vi "Write Permissions.vi"(8 "Error In":errorcluster) -> (0 "Error Out":errorcluster)   [LabVIEW 2018, in "Tests.lvlib" / "SFTP Attributes.lvlib"]
uses:
  SFTP Attributes.lvlib
  src/Toolkit/API/Typedefs/Permissions.ctl
  src/Toolkit/API/Typedefs/Modes.ctl
  src/Toolkit/API/SFTP Attributes/SFTP Attributes.lvclass/SFTP Attributes.ctl
  src/Toolkit/API/SSH/SSH.lvclass/SSH.ctl
  src/Toolkit/API/SSH/Utility/Read Shared Library.vi
  src/Toolkit/Support/Permissions to Bit Mask.vi
  src/Toolkit/Support/Bit Mask to Permissions.vi
  src/Toolkit/Support/Check Status.vi
  <vilib>/addons/_JKI Toolkits/Caraya/classes/Test/Test.lvclass
  <vilib>/addons/_JKI Toolkits/Caraya/classes/Assert/Assert.lvclass
  src/Toolkit/API/SFTP Attributes/SFTP Attributes.lvclass
  src/Toolkit/Toolkit.lvlib
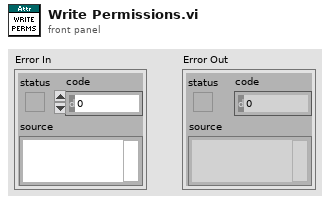
[diagram p1: front panel]
types:
  T1 = typedef "Toolkit.lvlib/Permissions.ctl" = cluster{"Owner":T2, "Group":T2, "Others":T2}
  T2 = typedef "Toolkit.lvlib/Modes.ctl" = cluster{"Read":bool, "Write":bool, "Execute":bool}
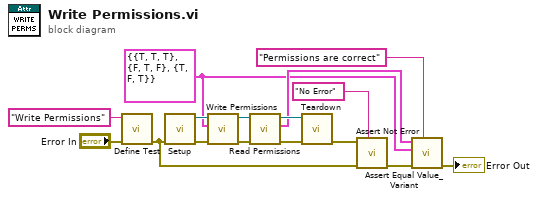
[diagram p0: block diagram]
diagram:
  w1 = T1 {"Owner"={"Read"=TRUE, "Write"=TRUE, "Execute"=TRUE}, "Group"={"Read"=FALSE, "Write"=TRUE, "Execute"=FALSE}, "Others"={"Read"=TRUE, "Write"=FALSE, "Execute"=TRUE}} ("Permissions")
  n1 = call <vilib>:"Define Test.vi"("error in (no error)"="Error In", "Label (VI Title)"="Write Permissions") -> ("error out"=w12:errorcluster)  [unwired: 9 in]
  n2 = call "Setup.vi"("Error In"=w12) -> ("Error Out"=w11:errorcluster, "SFTP Attributes"=w10:refnum<class "SFTP Attributes.lvclass">)  [unwired: 9 in]
  n3 = call "Write Permissions.vi"("Error In"=w11, "Permissions"=w1, "SFTP Attributes In"=w10) -> ("Error Out"=w6:errorcluster, "SFTP Attribute Out"=w9:refnum<class "SFTP Attributes.lvclass">)  [unwired: 7 in]
  n4 = call "Read Permissions.vi"("Error In"=w6, "SFTP Attributes In"=w9) -> ("Error Out"=w5:errorcluster, "Permissions"=w2:T1, "SFTP Attribute Out"=w7:refnum<class "SFTP Attributes.lvclass">)  [unwired: 7 in]
  n5 = call "Teardown.vi"("Error In"=w5, "SFTP Attributes"=w7) -> ("Error Out"=w8:errorcluster)  [unwired: 9 in]
  n6 = call <vilib>:"Assert Not Error.vi"("Label"="No Error", "error in (no error)"=w12, "Not Error?"=w8) -> ("error out"=w13:errorcluster)  [unwired: 8 in]
  n7 = call <vilib>:"Assert Equal Value_Variant.vi"("Label"="Permissions are correct", "error in (no error)"=w13, "Y"=w1, "X"=w2) -> ("error out"=→"Error Out":errorcluster)  [unwired: 7 in]
